vi "Get System Name.vi"(4 "Error In":errorcluster) -> (0 "Error Out":errorcluster, 2 "Ethernet Address":u32 format="%.0x", 3 "System Name":string)   [LabVIEW 2018]
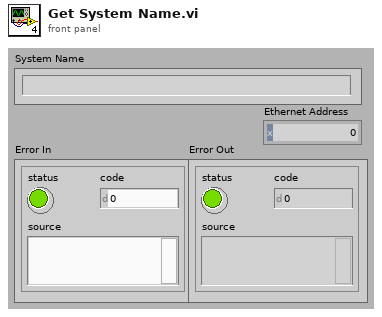
[diagram p1: front panel]
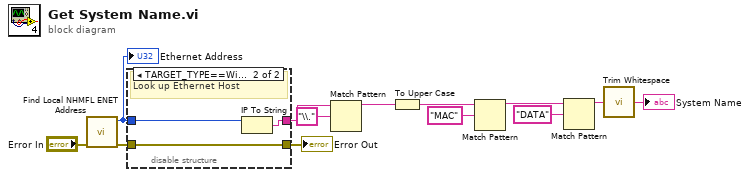
[diagram p0: block diagram]
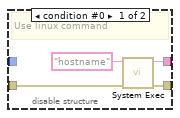
[diagram p2: hidden frame]
diagram:
  n1 = call "Find Local NHMFL ENET Address.vi"("error in (no error)"="Error In") -> ("error out"=w2:errorcluster, "Ethernet Address"=w3:u32)  [unwired: 9 in]
  "Ethernet Address" <- w3
  n2 = disable-structure shown="TARGET_TYPE==Windows" {
    disable-tunnel: w2 -> [w17 w18]
    disable-tunnel: [w15 w18] -> w1
    disable-tunnel: [w14 w20] -> w5
    disable-tunnel: w3 -> [_ w19]
    frame condition #0 {
      # "Use linux command"
      n3 = call <vilib>:"System Exec.vi"("error in (no error)"=w17, "command line"="hostname") -> ("error out"=w15:errorcluster, "standard output"=w14:string)  [unwired: 6 in, 2 out]
    }
    frame condition #1 (active) {
      # "Look up Ethernet Host"
      n4 = IP To String(2:w19) -> (0:w20:string)  [unwired: 1 in]
    }
  }
  "Error Out" <- w1
  n5 = Match Pattern(string=w5, regular expression="\\.") -> (before substring=w4:string)  [unwired: 1 in, 3 out]
  n6 = To Upper Case(1:w4) -> (0:w8:string)
  n7 = Match Pattern(string=w8, regular expression="MAC") -> (before substring=w10:string)  [unwired: 1 in, 3 out]
  n8 = Match Pattern(string=w10, regular expression="DATA") -> (before substring=w9:string)  [unwired: 1 in, 3 out]
  n9 = call <vilib>:"Trim Whitespace.vi"("string"=w9) -> ("trimmed string"=→"System Name":string)  [unwired: 1 in]
